vi "Refresh Control.vi"(8 "error in":errorcluster, 11 "PowerSupply in":refnum<class "PowerSupply.lvclass">) -> (0 "error out":errorcluster, 3 "PowerSupply out":refnum<class "PowerSupply.lvclass">)   [LabVIEW 2019, in "PowerSupply.lvlib" / "PowerSupply.lvclass"]
uses:
  Library/PowerSupply.lvclass
  Library/PowerSupply.lvclass/PowerSupply.ctl
  Accessors/Read Settings_Ref.vi
  Accessors/Read Settings.vi
  Accessors/Write Settings_Ref.vi
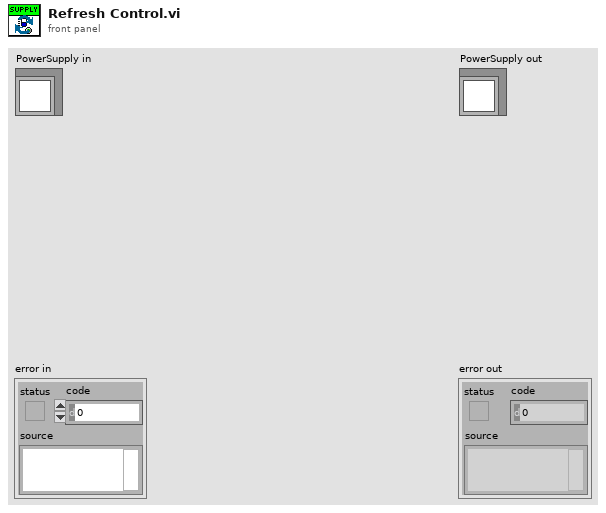
[diagram p1: front panel]
types:
  T1 = typedef "PowerSupply.lvlib/PowerSupply.lvclass/Settings.ctl" = cluster{"Voltage":dbl, "Current":dbl, "Output":bool, "OverVolt_Protect":dbl, "OverCurrent_Protect":dbl, "OVP":bool, "OCP":bool, "Interlock":bool, "Volt_Ramp":dbl, "Current_Ramp":dbl, "Sense Point":T2, "OCP Mode":T3, "Sharing":bool}
  T2 = typedef "PowerSupply.lvlib/PowerSupply.lvclass/Sense Point.ctl" = enum16{"Local", "Remote"}
  T3 = typedef "PowerSupply.lvlib/PowerSupply.lvclass/OCP Mode.ctl" = enum16{"Shutdown", "Foldback"}
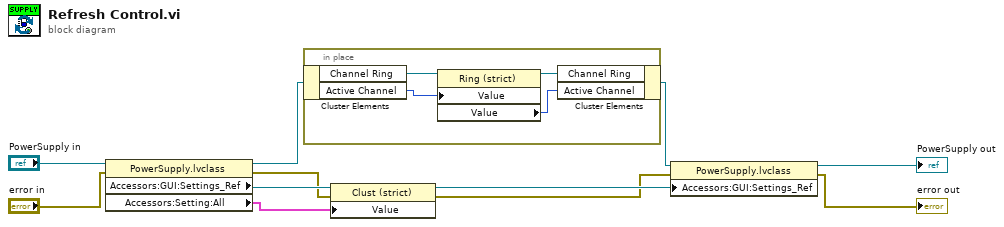
[diagram p0: block diagram]
diagram:
  n1 = property class="PowerSupply.lvclass"(reference="PowerSupply in", error in="error in") -> (reference out=w2:refnum<class "PowerSupply.lvclass">, error out=w8:errorcluster, "Accessors:GUI:Settings_Ref"=w10:refnum<vi>, "Accessors:Setting:All"=w9:T1)
  n2 = in-place {
    n3 = in-place-cluster #1(w2) -> ("Channel Ring"=w15:refnum<vi>, "Active Channel"=w13:u32)
    n4 = property class="Ring (strict)"(reference=w15, "Value"=w13) -> (reference out=w14:refnum<vi>, "Value"=w12:u16)  [unwired: 1 in, 1 out]
    n5 = in-place-cluster #1("Channel Ring"=w14, "Active Channel"=w12) -> (w1:refnum<class "PowerSupply.lvclass">)
  }
  n6 = property class="Clust (strict)"(reference=w10, error in=w8, "Value"=w9) -> (reference out=w6:refnum<vi>, error out=w5:errorcluster)
  n7 = property class="PowerSupply.lvclass"(reference=w1, error in=w5, "Accessors:GUI:Settings_Ref"=w6) -> (reference out=→"PowerSupply out":refnum<class "PowerSupply.lvclass">, error out=→"error out":errorcluster)
